vi "Day12-2.vi"() -> ()   [LabVIEW 2021]
panel:
  out "finished paths":i32
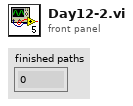
[diagram p1: front panel]
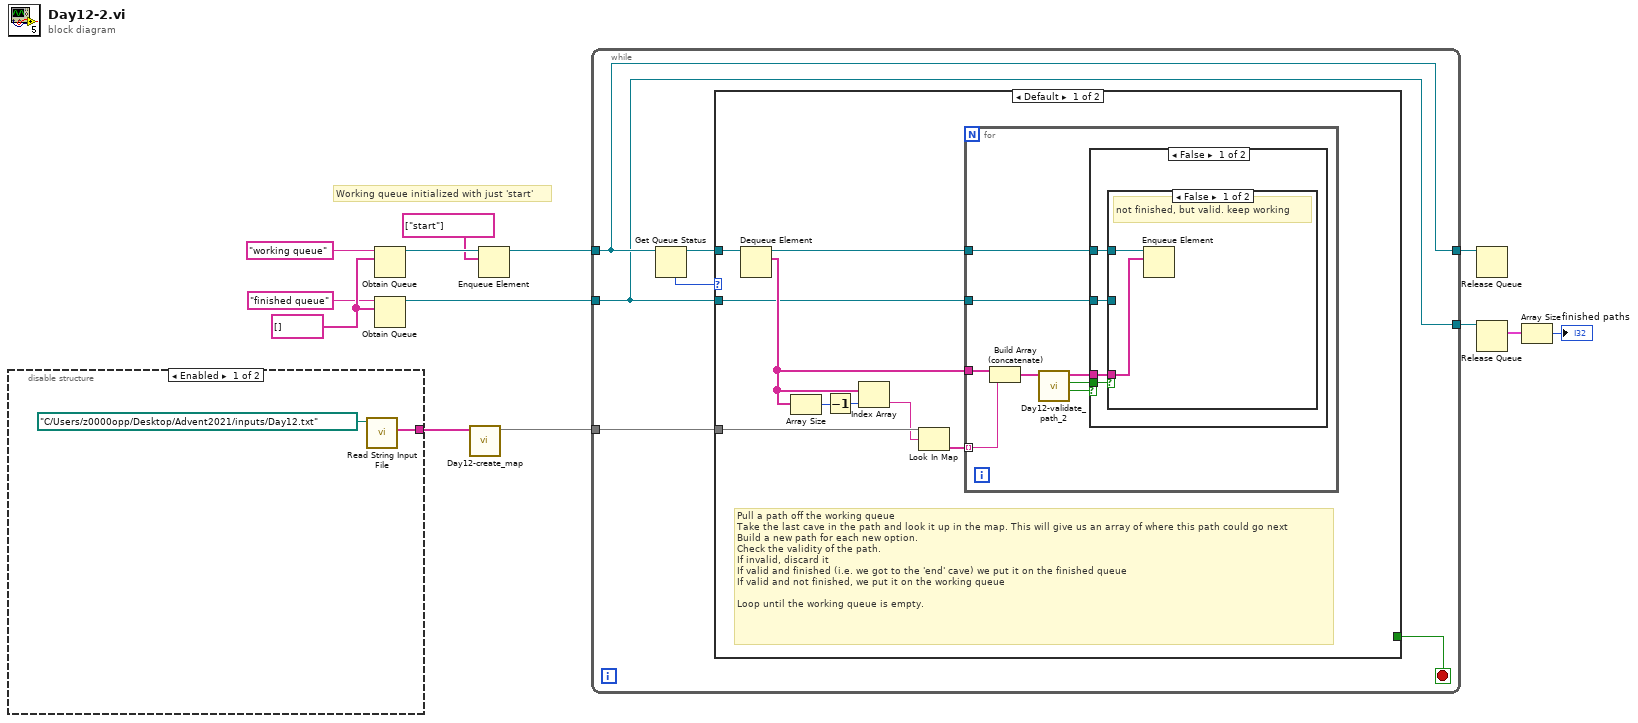
[diagram p0: block diagram]
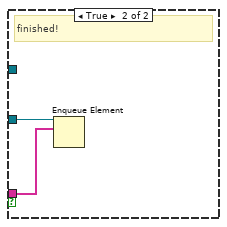
[diagram p2: hidden frame]
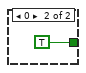
[diagram p4: hidden frame]
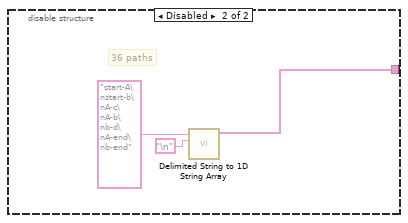
[diagram p5: hidden frame]
diagram:
  w10 = string[] []
  # "Working queue initialized with just 'start'"
  n1 = disable-structure shown="Enabled" {
    disable-tunnel: [w14 w16] -> w13
    frame Enabled {
      n2 = call "Read String Input File.vi"("file path (dialog if empty)"=path "C:/Users/z0000opp/Desktop/Advent2021/inputs/Day12.txt") -> ("input values"=w14:string[])  [unwired: 10 in]
    }
    frame Disabled {
      # "36 paths"
      n3 = call <vilib>:"Delimited String to 1D String Array.vi"("delimiter"="\n", "delimited string"="start-A\nstart-b\nA-c\nA-b\nb-d\nA-end\nb-end") -> ("string array"=w16:string[])  [unwired: 9 in]
    }
  }
  n4 = Obtain Queue(name (unnamed)="working queue", element data type=w10) -> (queue out=w12:refnum<queue>)  [unwired: 3 in, 2 out]
  n5 = Obtain Queue(name (unnamed)="finished queue", element data type=w10) -> (queue out=w5:refnum<queue>)  [unwired: 3 in, 2 out]
  n6 = call "Day12-create_map.vi"("string array"=w13) -> ("Map"=w7:map{string, string[]})  [unwired: 10 in]
  n7 = Enqueue Element(queue=w12, element=string[] ["start"]) -> (queue out=w6:refnum<queue>)  [unwired: 2 in, 2 out]
  n8 = while {
    tunnel: w7 -> [w21]
    tunnel: w6 -> [w20]
    tunnel: w5 -> [w19]
    tunnel: [w20] -> w4
    tunnel: [w19] -> w3
    stop <- w23 stop-if-true
    n9 = Get Queue Status(queue=w20) -> (queue out=w22:refnum<queue>, # elements in queue=w24:i32)  [unwired: 2 in, 6 out]
    n10 = case shown="Default" w24 {
      tunnel: [_ TRUE] -> w23
      tunnel: w22 -> [w33 _]
      tunnel: w19 -> [w25 _]
      tunnel: w21 -> [w30 _]
      frame Default {
        # "Pull a path off the working queue\nTake the last cave in the path and look it up in the map. This will give us an array of where this path could go next\nBuild a new path for each new option.\nCheck the validity of the path.\nIf invalid, discard it\nIf valid and finished (i.e. we got to the 'end' cave) we put it on the finished queue\nIf valid and not finished, we put it on the working queue\n\nLoop until the working queue is empty."
        n11 = Dequeue Element(queue=w33) -> (queue out=w26:refnum<queue>, element=w28:string[])  [unwired: 2 in, 2 out]
        n12 = Array Size(array=w28) -> (size(s)=w32:i32)
        n13 = Decrement(x=w32) -> (x-1=w31:i32)
        n14 = Index Array(array=w28, index=w31) -> (element=w29:string)
        n15 = Look In Map(map=w30, key=w29) -> (value=w27:string[])  [unwired: 1 in, 1 out]
        n16 = for {
          tunnel: w28 -> [w41]
          tunnel: w27 -> [w40] mode=indexing
          tunnel: w26 -> [w34]
          tunnel: w25 -> [w35]
          n17 = Build Array (concatenate)(w41, w40) -> (w39:string[])
          n18 = call "Day12-validate_path_2.vi"("Path"=w39) -> ("invalid?"=w38:bool, "finshed?"=w36:bool, "Path out"=w37:string[])  [unwired: 8 in]
          n19 = case shown="False" w38 {
            tunnel: w37 -> [w43 _]
            tunnel: w36 -> [w45 _]
            tunnel: w35 -> [w44 _]
            tunnel: w34 -> [w42 _]
            frame False {
              n20 = case shown="False" w45 {
                tunnel: w44 -> [_ w49]
                tunnel: w43 -> [w46 w48]
                tunnel: w42 -> [w47 _]
                frame False {
                  # "not finished, but valid. keep working"
                  n21 = Enqueue Element(queue=w47, element=w46) -> ()  [unwired: 2 in, 3 out]
                }
                frame True {
                  # "finished!"
                  n22 = Enqueue Element(queue=w49, element=w48) -> ()  [unwired: 2 in, 3 out]
                }
              }
            }
            frame True {
              # "invalid, do nothing"
            }
          }
        }
      }
      frame 0 {
      }
    }
  }
  n23 = Release Queue(queue=w4) -> ()  [unwired: 2 in, 3 out]
  n24 = Release Queue(queue=w3) -> (remaining elements=w2:cluster{string[]}[])  [unwired: 2 in, 2 out]
  n25 = Array Size(array=w2) -> (size(s)=→"finished paths":i32)
